vi "Mask Buffer.vi"(1 "Write Data":T1={"Write Index"=0, "Write Element"=0, "Write?"=TRUE}, 7 "Read Address 0":i32, 11 "Read Address 1":i32) -> (8 "Output 0":i16, 15 "Output 1":i16)   [LabVIEW 2014]
doc: "<b> BRAM Usage = 2 of Size 16,000 I15's </b>"
panel:
  # "Copyright 2014 Vidrio Technologies\nScanImage 5 software is licensed under the Apache License, Version 2.0 (the \"License\"); you may not use any files contained\nwithin the ScanImage 5 release except in compliance with the License. You may obtain a copy of the License at\n http://www.apache.org/licenses/LICENSE-2.0\nUnless required by applicable law or agreed to in writing, software distributed under the License is distributed on an\n\"AS IS\" BASIS, WITHOUT WARRANTIES OR CONDITIONS OF ANY KIND, either express or implied. See the License for the\n specific language governing permissions and limitations under the License."
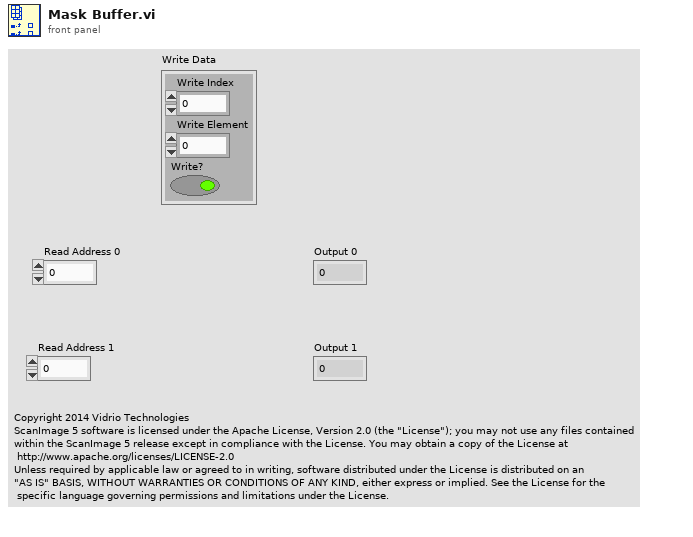
[diagram p1: front panel]
types:
  T1 = cluster{"Write Index":i32, "Write Element":i32, "Write?":bool}
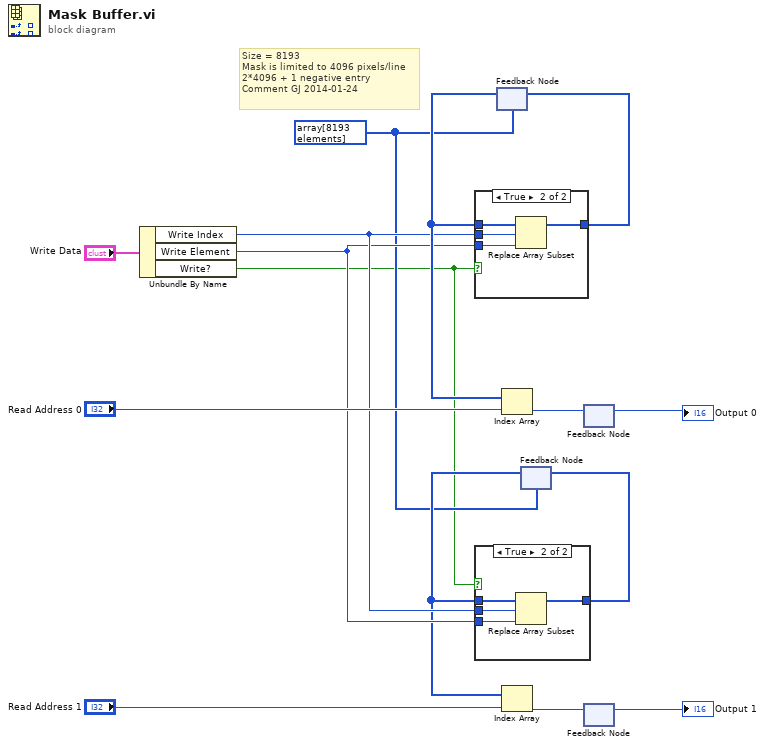
[diagram p0: block diagram]
diagram:
  w2 = i16[] array[8193 elements]
  # "Size = 8193\nMask is limited to 4096 pixels/line\n2*4096 + 1 negative entry\nComment GJ 2014-01-24"
  n1 = Unbundle By Name("Write Data") -> ("Write Index"=w9:i32, "Write Element"=w8:i32, "Write?"=w1:bool)
  n2 = feedback #1(w2) -> (w14:i16[])
  n3 = case shown="True" w1 {
    tunnel: [w16 w20] -> w15
    tunnel: w14 -> [w16 w19]
    tunnel: w9 -> [_ w18]
    tunnel: w8 -> [_ w17]
    frame False {
    }
    frame True {
      n4 = Replace Array Subset(array=w19, new element=w17, index=w18) -> (w20:i16[])
    }
  }
  n5 = feedback-in #1(w15) -> ()
  n6 = Index Array(array=w14, index="Read Address 0") -> (element=w12:i16)
  n7 = feedback #2(w2) -> (w5:i16[])
  n8 = case shown="True" w1 {
    tunnel: w9 -> [_ w25]
    tunnel: w8 -> [_ w24]
    tunnel: [w21 w23] -> w6
    tunnel: w5 -> [w21 w22]
    frame False {
    }
    frame True {
      n9 = Replace Array Subset(array=w22, new element=w24, index=w25) -> (w23:i16[])
    }
  }
  n10 = Index Array(array=w5, index="Read Address 1") -> (element=w4:i16)
  n11 = feedback-in #2(w6) -> ()
  n12 = feedback-in #3(w12) -> ()
  n13 = feedback #3() -> (→"Output 0":i16)  [unwired: 1 in]
  n14 = feedback #4() -> (→"Output 1":i16)  [unwired: 1 in]
  n15 = feedback-in #4(w4) -> ()
